vi "Create Pump.vi"(6 "Pump Name":string, 8 "error in (no error)":errorcluster, 11 "Worker in":refnum<class "Worker.lvclass">) -> (0 "error out":errorcluster, 3 "Worker out":refnum<class "Worker.lvclass">)   [LabVIEW 2023, in "Message Pump.lvclass"]
uses:
  Message Pump.lvclass
  <vilib>/addons/_Workers/Library/Classes/Worker/Worker.lvclass
  <vilib>/addons/_Workers/Library/Classes/Worker/Worker.lvclass/Worker.ctl
  Initialization Data.ctl
  <vilib>/addons/_Workers/Library/Classes/Message Queue/Message Queue.lvclass
  C:/Program Files (x86)/National Instruments/LabVIEW 2023/vi.lib/addons/_Workers/Library/Classes/Worker/Worker.lvclass
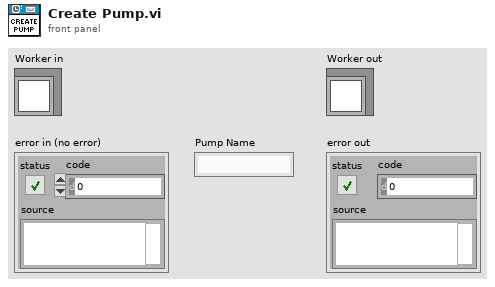
[diagram p1: front panel]
types:
  T1 = typedef "Message Pump.lvclass/Initialization Data.ctl" = cluster{"Caller Queue":refnum<class "Message Queue.lvclass">}
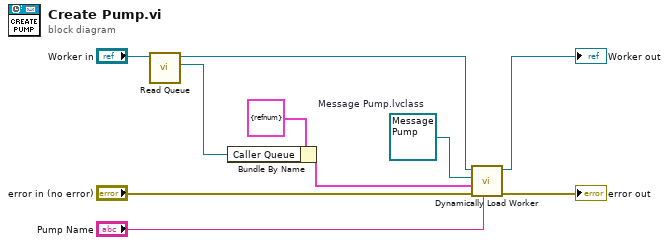
[diagram p0: block diagram]
diagram:
  w4 = refnum<class "Message Pump.lvclass"> refnum  # Message Pump.lvclass
  n1 = call <vilib>:"Read Queue.vi"("Worker"="Worker in") -> ("Message Queue out"=w2:refnum<class "Message Queue.lvclass">, "dup Worker out"=w1:refnum<class "Worker.lvclass">)  [unwired: 9 in]
  n2 = Bundle By Name(cluster=T1 {"Caller Queue"=refnum} ("Initialization Data"), "Caller Queue"=w2) -> (w3:T1)
  n3 = call <vilib>:"Dynamically Load Worker.vi"("Worker Alias"="Pump Name", "error in"="error in (no error)", "Initialization Data"=w3, "Worker to Dynamically Load"=w4, "Worker"=w1) -> ("error out"=→"error out":errorcluster, "dup Worker out"=→"Worker out":refnum<class "Worker.lvclass">)  [unwired: 3 in, 2 out]
